vi "Write Config to File.vi"(8 "error in (no error)":errorcluster, 11 "Macro in":refnum<class "Macro.lvclass">) -> (0 "error out":errorcluster, 3 "Macro out":refnum<class "Macro.lvclass">)   [LabVIEW 2020, in "MacroAssert.lvlib" / "Macro.lvclass"]
uses:
  Macro.lvclass
  Macro.lvclass/Macro.ctl
  <vilib>/Utility/config.llb/NI_LVConfig.lvlib
  <vilib>/Utility/config.llb/Write Key (I32).vi
  <vilib>/Utility/config.llb/Write Key (String).vi
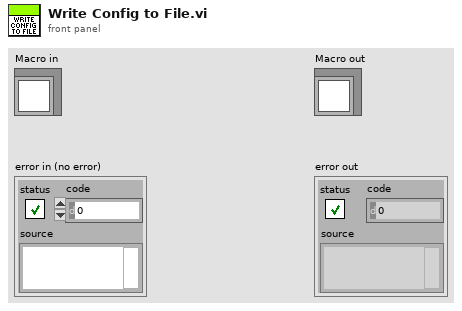
[diagram p1: front panel]
types:
  T1 = typedef "MacroAssert.lvlib/Macro Config V3.ctl" = cluster{"Schema Version":string, "Activation Type":enum32{"Hotkey", "Automatic"}, "N":i32, "Description":string, "Resolutions":cluster{"Width":i16, "Height":i16}[], "Date Created":timestamp, "Date Updated":timestamp}
  T2 = typedef "NI_LVConfig.lvlib/Config Data RefNum.ctl" = refnum<k1>
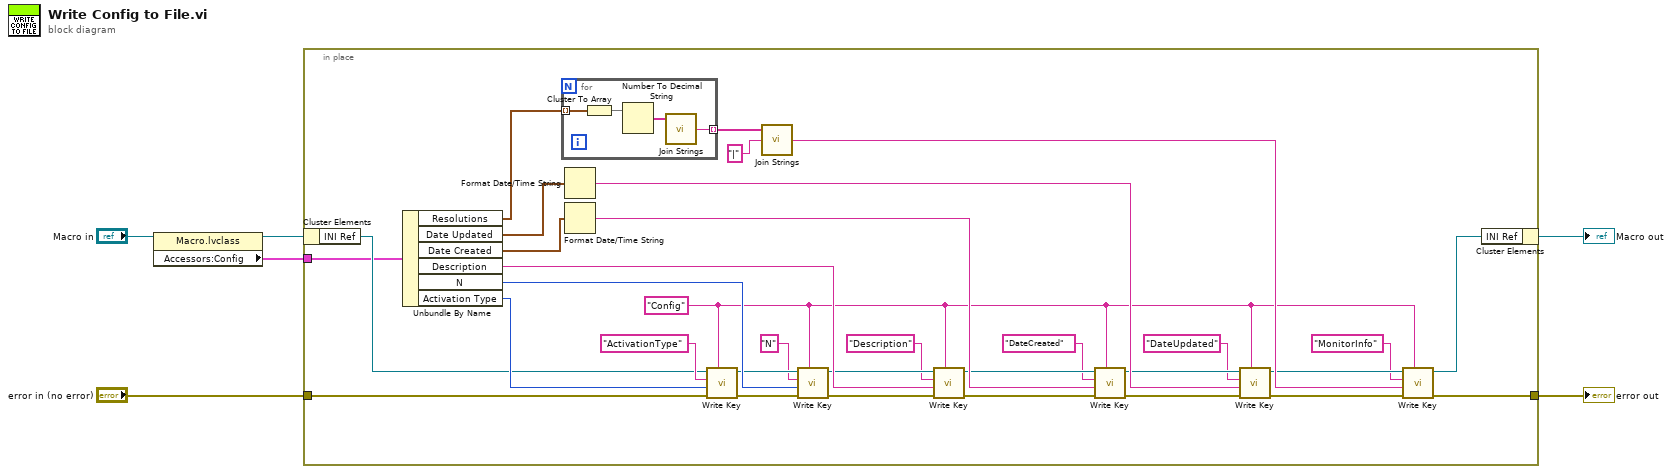
[diagram p0: block diagram]
diagram:
  n1 = property class="Macro.lvclass"(reference="Macro in") -> (reference out=w2:refnum<class "Macro.lvclass">, "Accessors:Config"=w1:T1)  [unwired: 1 in, 1 out]
  n2 = in-place {
    in-place-border: "error in (no error)" -> [w11]
    in-place-border: [w9] -> w4
    in-place-border: w1 -> [w7]
    w18 = "Config" ("section")
    n3 = in-place-cluster #1(w2) -> ("INI Ref"=w10:T2)
    n4 = Unbundle By Name(w7) -> ("Resolutions"=w36:cluster{"Width":i16, "Height":i16}[], "Date Updated"=w35:timestamp, "Date Created"=w34:timestamp, "Description"=w32:string, "N"=w31:i32, "Activation Type"=w30:enum32{"Hotkey", "Automatic"})
    n5 = for {
      tunnel: w36 -> [w43] mode=indexing
      tunnel: [w40] -> w33 mode=indexing
      n6 = Cluster To Array(cluster=w43) -> (array=w42:i16[])
      n7 = Number To Decimal String(number=w42) -> (decimal integer string=w41:string[])  [unwired: 1 in]
      n8 = call <vilib>:"Join Strings.vi"("Strings In"=w41) -> ("String"=w40:string)  [unwired: 2 in]
    }
    n9 = Format Date/Time String(seconds (now)=w35) -> (date/time string=w38:string)  [unwired: 2 in]
    n10 = Format Date/Time String(seconds (now)=w34) -> (date/time string=w37:string)  [unwired: 2 in]
    n11 = call-poly <vilib>:"Write Key.vi"("section"=w18, "error in (no error)"=w11, "value"=w30, "key"="ActivationType", "refnum"=w10) -> ("error out"=w25:errorcluster, "refnum out"=w20:T2)  [unwired: 4 in, 1 out]
    n12 = call <vilib>:"Join Strings.vi"("Separator (,)"="|", "Strings In"=w33) -> ("String"=w39:string)  [unwired: 1 in]
    n13 = call-poly <vilib>:"Write Key.vi"("section"=w18, "error in (no error)"=w25, "value"=w31, "key"="N", "refnum"=w20) -> ("error out"=w26:errorcluster, "refnum out"=w21:T2)  [unwired: 4 in, 1 out]
    n14 = call-poly <vilib>:"Write Key.vi"("section"=w18, "error in (no error)"=w26, "value"=w32, "key"="Description", "refnum"=w21) -> ("error out"=w27:errorcluster, "refnum out"=w22:T2)  [unwired: 4 in, 1 out]
    n15 = call-poly <vilib>:"Write Key.vi"("section"=w18, "error in (no error)"=w27, "value"=w37, "key"="DateCreated", "refnum"=w22) -> ("error out"=w28:errorcluster, "refnum out"=w23:T2)  [unwired: 4 in, 1 out]
    n16 = call-poly <vilib>:"Write Key.vi"("section"=w18, "error in (no error)"=w28, "value"=w38, "key"="DateUpdated", "refnum"=w23) -> ("error out"=w29:errorcluster, "refnum out"=w24:T2)  [unwired: 4 in, 1 out]
    n17 = call-poly <vilib>:"Write Key.vi"("section"=w18, "error in (no error)"=w29, "value"=w39, "key"="MonitorInfo", "refnum"=w24) -> ("error out"=w9:errorcluster, "refnum out"=w8:T2)  [unwired: 4 in, 1 out]
    n18 = in-place-cluster #1("INI Ref"=w8) -> (→"Macro out":refnum<class "Macro.lvclass">)
  }
  "error out" <- w4
